vi "Write Sim Axis Data.vi"(8 "error in (no error)":errorcluster, 10 "Sim Axis Data":T1, 11 "Parent SIM Motion Controller in":refnum<class "Parent SIM Motion Controller.lvclass">) -> (0 "error out":errorcluster, 3 "Parent SIM Motion Controller out":refnum<class "Parent SIM Motion Controller.lvclass">)   [LabVIEW 2022 SP3, in "Parent SIM Motion Controller.lvclass"]
uses:
  Parent SIM Motion Controller.lvclass
  Axis Data.ctl
  Axis Parameters.ctl
  Axis Settings.ctl
  Parent SIM Motion Controller.lvclass/Parent SIM Motion Controller.ctl
  Homing Status.ctl
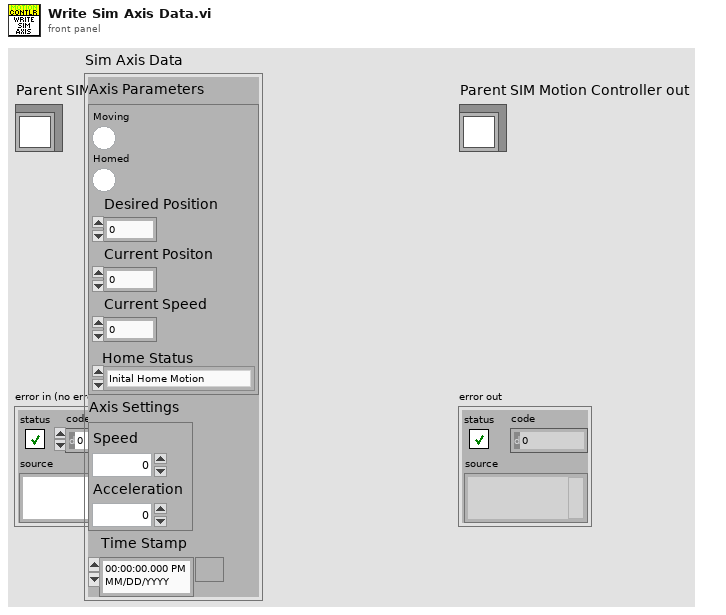
[diagram p1: front panel]
types:
  T1 = typedef "Parent SIM Motion Controller.lvclass/Axis Data.ctl" = cluster{"Axis Parameters":T2, "Axis Settings":T4, "Time Stamp":timestamp}
  T2 = typedef "Parent SIM Motion Controller.lvclass/Axis Parameters.ctl" = cluster{"Moving":bool, "Homed":bool, "Desired Position":dbl, "Current Positon":dbl, "Current Speed":dbl, "Home Status":T3}
  T3 = typedef "Parent SIM Motion Controller.lvclass/Homing Status.ctl" = enum16{"Inital Home Motion", "Final Home Motion"}
  T4 = typedef "Parent SIM Motion Controller.lvclass/Axis Settings.ctl" = cluster{"Speed":dbl, "Acceleration":dbl}
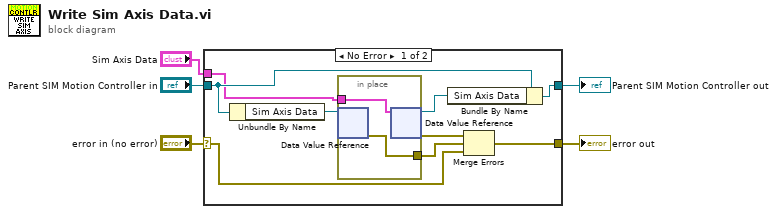
[diagram p0: block diagram]
diagram:
  n1 = case shown="No Error" "error in (no error)" {
    selector: "error in (no error)" -> [w7 w17]
    tunnel: [w6 w17] -> w4
    tunnel: [w14 w18] -> w2
    tunnel: "Parent SIM Motion Controller in" -> [w13 w18]
    tunnel: "Sim Axis Data" -> [w11 _]
    frame No Error {
      n2 = Unbundle By Name(w13) -> ("Sim Axis Data"=w12:refnum<data-value>)
      n3 = in-place {
        in-place-border: w11 -> [w16]
        in-place-border: [w15] -> w9
        n4 = in-place-dvr #1(w12) -> (w15:errorcluster)  [unwired: 1 out]
        n5 = in-place-dvr #1(w16) -> (w10:refnum<data-value>, w8:errorcluster)
      }
      n6 = Bundle By Name(cluster=w13, "Sim Axis Data"=w10) -> (w14:refnum<class "Parent SIM Motion Controller.lvclass">)
      n7 = Merge Errors(w8, w9, w7) -> (w6:errorcluster)
    }
    frame Error {
    }
  }
  "error out" <- w4
  "Parent SIM Motion Controller out" <- w2
